vi "mclamp_set_Iholding_01.vi"(8 "error in (no error)":errorcluster, 9 "set holding (pA)":dbl, 10 "Error in":i32, 11 "Multiclamp Handle Out":u32) -> (0 "error out":errorcluster, 2 "error out":i32)   [LabVIEW 2019]
uses:
  patcherBot_software_all/patcherBot_Software/patcherBot/AxMultiClampMsg.dll
panel:
  out "ModeConstant":dbl
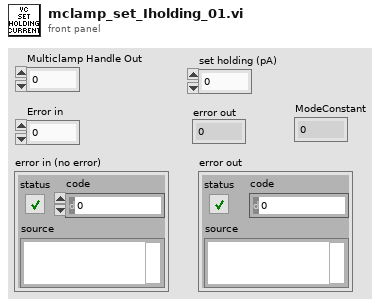
[diagram p1: front panel]
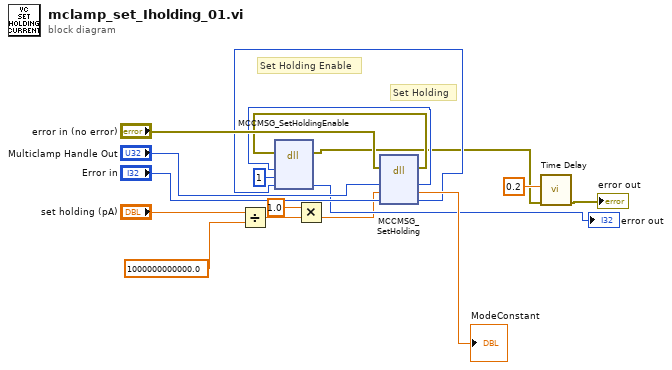
[diagram p0: block diagram]
diagram:
  # "Set Holding Enable"
  # "Set Holding"
  n1 = Divide(x="set holding (pA)", y=1000000000000.0) -> (x/y=w14:dbl)
  n2 = Multiply(x=1.0, y=w14) -> (x*y=w2:dbl)
  n3 = dll-call lib="C:/Users/might/Dropbox (GaTech)/patcherBot_software_all/patcherBot_Software/patcherBot/AxMultiClampMsg.dll" fn="MCCMSG_SetHolding"(error in="error in (no error)", "handle"="Multiclamp Handle Out", "ModeConstant"=w2, "error"="Error in") -> (error out=w9:errorcluster, "handle"=w6:u32, "ModeConstant"=→"ModeConstant":dbl, "error"=w5:i32)  [unwired: 3 in, 1 out]
  n4 = dll-call lib="C:/Users/might/Dropbox (GaTech)/patcherBot_software_all/patcherBot_Software/patcherBot/AxMultiClampMsg.dll" fn="MCCMSG_SetHoldingEnable"(error in=w9, "handle"=w6, "ModeConstant"=1, "error"=w5) -> (error out=w3:errorcluster, "error"=→"error out":i32)  [unwired: 5 in, 1 out]
  n5 = call "Time Delay"("error in (no error)"=w3, "Delay Time (s)"=0.2) -> ("error out"=→"error out":errorcluster)  [unwired: 9 in]
